vi "matlab test.vi"() -> ()   [LabVIEW 2020]
panel:
  out "2-D Array of Complex":cdb[][](array[numeric])
  in  "1-D Array of Complex":cdb[](array[numeric])
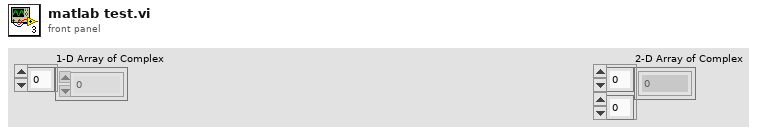
[diagram p1: front panel]
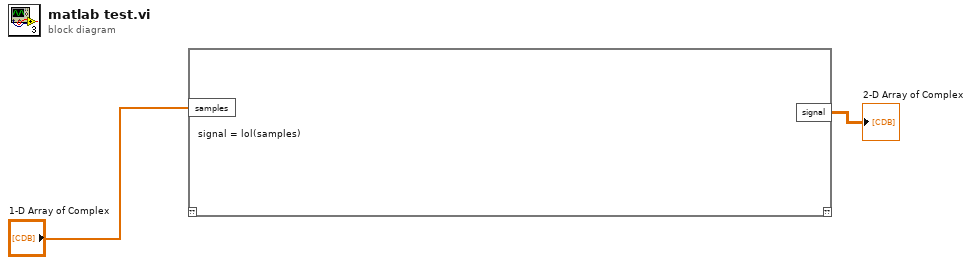
[diagram p0: block diagram]
diagram:
  n1 = script code="signal = lol(samples)"("samples"="1-D Array of Complex") -> ("signal"=→"2-D Array of Complex":cdb[][])  [unwired: 1 in, 1 out]
